vi "TDMS Find MN-SN Path.vi"(8 "error in (no error)":errorcluster, 9 "Serial Number":string, 10 "Model Number":string) -> (0 "error out":errorcluster, 1 "Found?":bool, 2 "MN-SN Path":path)   [LabVIEW 2011]
uses:
  DataFinder/Datafinder Query.ctl
  DataFinder/eSearch Types.ctl
  DataFinder/DataFinder Comparisons.ctl
  DIAdem/lib/DIAdem Query Queue.ctl
  Summitek EXT/OpenG EXT/file/file.llb/File Exists - Scalar__ogtk.vi
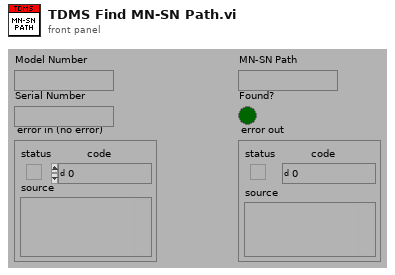
[diagram p1: front panel]
types:
  T1 = typedef "DIAdem Query Queue.ctl" = cluster{"UserName":string, "Search Parameters":T2[], "eSearch Type":T3, "Query Name (vbs)":string, "Response queue name":string, "Logic String":string}
  T2 = typedef "Datafinder Query.ctl" = cluster{"eSearch Types":T3, "Property Name":string, "DataFinder Comparisons":T4, "Property Value":string}
  T3 = typedef "eSearch Types.ctl" = enum16{"eSearchFile", "eSearchChannelGroup", "eSearchChannel"}
  T4 = typedef "DataFinder Comparisons.ctl" = enum16{"=", "<>", "<", "<=", ">", ">="}
  T5 = typedef "DIAdem Query Result.ctl" = cluster{"Results":string[][], "# of Items":i32, "Data Returned?":bool, "Result TDM":path, "Timed Out?":bool}
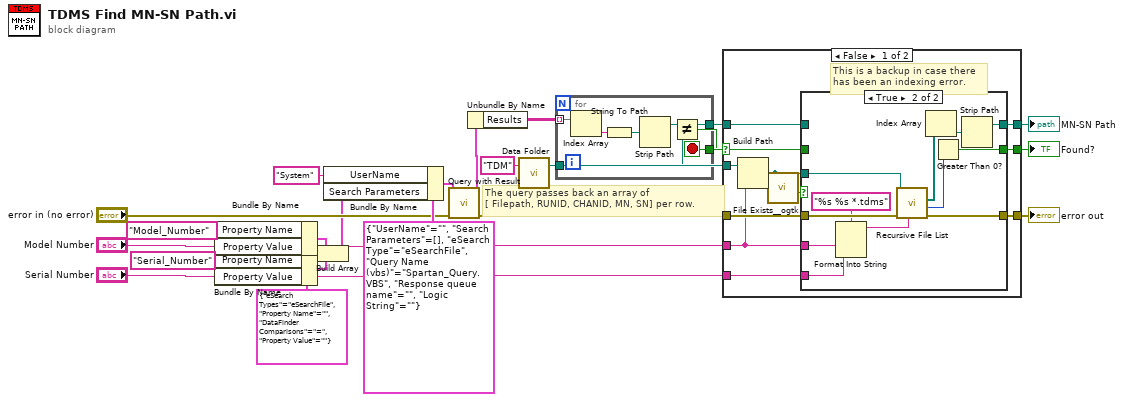
[diagram p0: block diagram]
diagram:
  w17 = T2 {"eSearch Types"=enum."eSearchFile", "Property Name"="", "DataFinder Comparisons"=enum."=", "Property Value"=""} ("Data Finder Parameters")
  # "The query passes back an array of\n[ Filepath, RUNID, CHANID, MN, SN] per row."
  n1 = Bundle By Name(cluster=w17, "Property Name"="Model_Number", "Property Value"="Model Number") -> (w19:T2)
  n2 = Bundle By Name(cluster=w17, "Property Name"="Serial_Number", "Property Value"="Serial Number") -> (w18:T2)
  n3 = Build Array(w19, w18) -> (w13:T2[])
  n4 = Bundle By Name(cluster=T1 {"UserName"="", "Search Parameters"=[], "eSearch Type"=enum."eSearchFile", "Query Name (vbs)"="Spartan_Query.VBS", "Response queue name"="", "Logic String"=""} ("Query Parameter Data"), "UserName"="System", "Search Parameters"=w13) -> (w14:T1)
  n5 = call "Query with Result.vi"("error in (no error)"="error in (no error)", "Query Parameter Data"=w14) -> ("error out"=w9:errorcluster, "Query Return Data"=w12:T5)  [unwired: 1 in, 7 out]
  n6 = Unbundle By Name(w12) -> ("Results"=w11:string[][])
  n7 = call "Data Folder.vi"("Relative Path (\"\" - Folder)"="TDM" ("Relative Path (\"\" - Folder)")) -> ("Data Folder"=w3:path)  [unwired: 2 in]
  n8 = for {
    tunnel: w11 -> [w25] mode=indexing
    tunnel: w3 -> [w28]
    tunnel: [w27] -> w5
    tunnel: [w26] -> w7
    stop <- w26 stop-if-true
    n9 = Index Array(array=w25) -> (element=w24:string)  [unwired: 1 in]
    n10 = String To Path(string=w24) -> (path=w23:path)
    n11 = Strip Path(path=w23) -> (stripped path=w27:path)  [unwired: 1 out]
    n12 = Not Equal?(x=w27, y=w28) -> (x != y?=w26:bool)
  }
  n13 = case shown="False" w7 {
    selector: w7 -> [w32 w57]
    tunnel: w9 -> [w39 w56]
    tunnel: [w35 w56] -> w8
    tunnel: [w31 w57] -> w6
    tunnel: w5 -> [w34 w55]
    tunnel: [w33 w55] -> w4
    tunnel: "Model Number" -> [w30 _]
    tunnel: "Serial Number" -> [w29 _]
    tunnel: w3 -> [w38 _]
    frame False {
      # "This is a backup in case there\nhas been an indexing error."
      n14 = Build Path(base path=w38, name or relative path=w30) -> (appended path=w37:path)
      n15 = call-poly "File Exists__ogtk.vi"("file path"=w37) -> ("exists"=w36:bool)  [unwired: 6 in, 1 out]
      n16 = case shown="True" w36 {
        tunnel: w39 -> [w42 w54]
        tunnel: w37 -> [_ w53]
        tunnel: [w42 w52] -> w35
        tunnel: w34 -> [w41 _]
        tunnel: [w41 w44] -> w33
        tunnel: w32 -> [w40 _]
        tunnel: [w40 w46] -> w31
        tunnel: w30 -> [_ w50]
        tunnel: w29 -> [_ w49]
        frame False {
        }
        frame True {
          n17 = Format Into String(format string="%s %s *.tdms", w50, w49) -> (resulting string=w48:string)  [unwired: 2 in, 1 out]
          n18 = call <vilib>:"Recursive File List.vi"("pattern"=w48, "error in (no error)"=w54, "Folder Path"=w53) -> ("error out"=w52:errorcluster, "Number of Files"=w47:i32, "All Files in Dir"=w43:path[])  [unwired: 4 in, 2 out]
          n19 = Index Array(array=w43) -> (element=w45:path)  [unwired: 1 in]
          n20 = Greater Than 0?(x=w47) -> (x > 0?=w46:bool)
          n21 = Strip Path(path=w45) -> (stripped path=w44:path)  [unwired: 1 out]
        }
      }
    }
    frame True {
    }
  }
  "error out" <- w8
  "MN-SN Path" <- w4
  "Found?" <- w6
